vi "cal_error.vi"(9 "X":dbl[](array[numeric]), 11 "Cal data":dbl[][](array[numeric])) -> (0 "Residuals":dbl[](array[numeric]) format="%#_4p", 2 "f(X)":dbl)   [LabVIEW 2014]
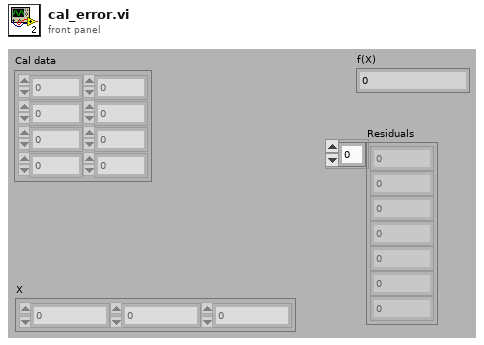
[diagram p1: front panel]
types:
  T1 = typedef "calibration.ctl" = cluster{"Ks":dbl[][], "r bias":dbl}
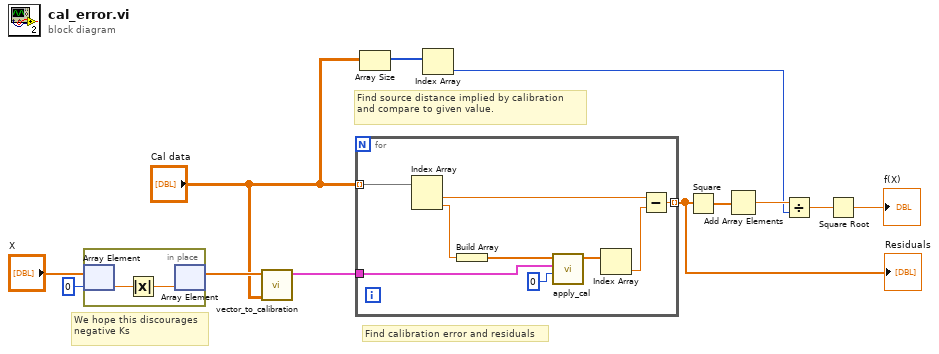
[diagram p0: block diagram]
diagram:
  # "We hope this discourages negative Ks"
  # "Find calibration error and residuals"
  # "Find source distance implied by calibration and compare to given value."
  n1 = in-place {
    n2 = in-place-array #1("X", 0) -> (w14:dbl)
    n3 = Absolute Value(x=w14) -> (abs(x)=w13:dbl)
    n4 = in-place-array #1(w13) -> (w4:dbl[])  [unwired: 1 out]
  }
  n5 = call "vector_to_calibration.vi"("Cal data"="Cal data", "minimum"=w4) -> ("Calibration out"=w3:T1)  [unwired: 9 in]
  n6 = for {
    tunnel: "Cal data" -> [w18] mode=indexing
    tunnel: [w23] -> w8 mode=indexing
    tunnel: w3 -> [w16]
    n7 = Index Array(array=w18) -> (element #1=w22:dbl, element #2=w17:dbl)  [unwired: 2 in]
    n8 = Build Array(w17) -> (w21:dbl[])
    n9 = call "apply_cal.vi"("High/low index"=0, "Calibration"=w16, "V"=w21) -> ("r"=w20:dbl[])  [unwired: 8 in]
    n10 = Index Array(array=w20) -> (element=w19:dbl)  [unwired: 1 in]
    n11 = Subtract(x=w22, y=w19) -> (x-y=w23:dbl)
  }
  "Residuals" <- w8
  n12 = Array Size(array="Cal data") -> (size(s)=w7:i32[])
  n13 = Index Array(array=w7) -> (element=w6:i32)  [unwired: 1 in]
  n14 = Square(x=w8) -> (x^2=w10:dbl[])
  n15 = Add Array Elements(numeric array=w10) -> (sum=w9:dbl)
  n16 = Divide(x=w9, y=w6) -> (x/y=w11:dbl)
  n17 = Square Root(x=w11) -> (sqrt(x)=→"f(X)":dbl)
